vi "GetCurrentViPath.vi"(1 "PathIn":path) -> (0 "CurrentViPath":path)   [LabVIEW 2013]
uses:
  SourceCode/GlobalValue.vi
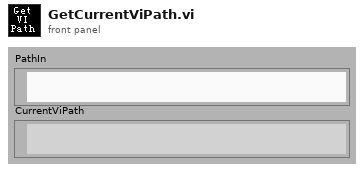
[diagram p1: front panel]
types:
  T1 = enum32{"invalid app kind", "Development System", "Run Time System", "Student Edition", "Embedded LabVIEW", "Evaluation", "Custom"}
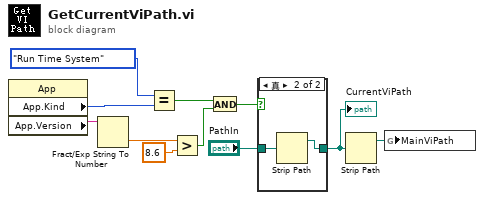
[diagram p0: block diagram]
diagram:
  n1 = property class="App"() -> ("App.Kind"=w6:T1, "App.Version"=w7:string)  [unwired: 2 in, 2 out]
  n2 = Fract/Exp String To Number(string=w7) -> (number=w8:dbl)  [unwired: 4 out]
  n3 = Equal?(x=T1."Run Time System" ("y"), y=w6) -> (x = y?=w10:bool)
  n4 = Greater?(x=w8, y=8.6) -> (0:w11:bool)
  n5 = And(x=w10, y=w11) -> (x .and. y?=w4:bool)
  n6 = case shown="真" w4 {
    tunnel: [w12 w14] -> w2
    tunnel: "PathIn" -> [w12 w13]
    frame False {
    }
    frame True {
      n7 = Strip Path(path=w13) -> (stripped path=w14:path)  [unwired: 1 out]
    }
  }
  "CurrentViPath" <- w2
  n8 = Strip Path(path=w2) -> (stripped path=w1:path)  [unwired: 1 out]
  n9 = global write "GlobalValue.vi" "MainViPath"(w1) -> ()
